vi "test_DiscoveryServiceNotRunning_LaunchDiscoveryService_DiscoveryServiceStarted.vi"(8 "error in":errorcluster) -> (0 "error out":errorcluster, 2 "result":string, 3 "pass":bool)   [LabVIEW 2020, in "MeasurementServerTests.lvlib" / "Discovery Tests.lvlib"]
uses:
  Discovery Tests.lvlib
  Runtime/MeasurementLink Discovery V1/MeasurementLink Discovery V1.lvlib
  MeasurementServerTests.lvlib
  Runtime/MeasurementLink Discovery V1/TypeDefs/gRPC Client Cache FGV Action.ctl
  Runtime/MeasurementLink Discovery Client/MeasurementLink Discovery Client.lvlib
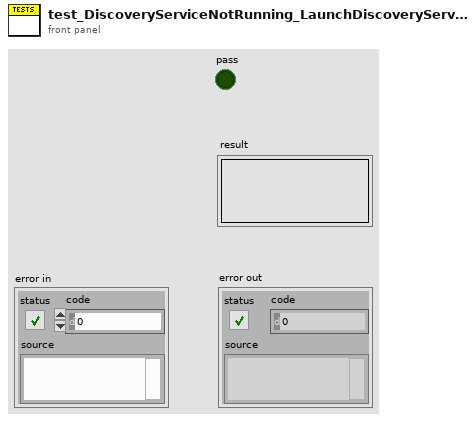
[diagram p1: front panel]
types:
  T1 = typedef "MeasurementLink Discovery V1.lvlib/gRPC Client Cache FGV Action.ctl" = enum16{"Get Client", "Recreate Client"}
  T2 = typedef "grpc-lvsupport-release.lvlib/grpcId.ctl" = u64
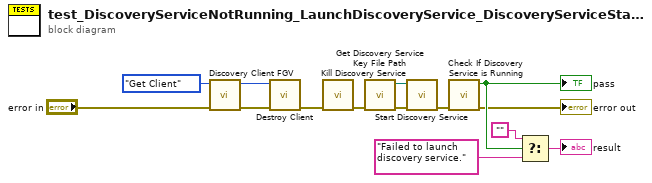
[diagram p0: block diagram]
diagram:
  n1 = call "Discovery Client FGV.vi"("error in"="error in", "action"=gRPC_Client_Cache_FGV_Action."Get Client") -> ("error out"=w4:errorcluster, "grpc client id"=w3:T2)  [unwired: 7 in, 1 out]
  n2 = call "Destroy Client.vi"("error in"=w4, "gRPC ID"=w3) -> ("error out"=w1:errorcluster)  [unwired: 9 in]
  n3 = call "Kill Discovery Service.vi"("error in"=w1) -> ("error out"=w13:errorcluster)  [unwired: 10 in]
  n4 = call "Get Discovery Service Key File Path.vi"("error in"=w13) -> ("error out"=w14:errorcluster, "key file path"=w9:path)  [unwired: 9 in]
  n5 = call "Start Discovery Service.vi"("error in"=w14, "key file path"=w9) -> ("error out"=w8:errorcluster)  [unwired: 9 in]
  n6 = call "Check If Discovery Service is Running.vi"("error in"=w8) -> ("error out"=→"error out":errorcluster, "discovery service running?"=w7:bool)  [unwired: 9 in]
  "pass" <- w7
  n7 = Select(t="", s=w7, f="Failed to launch discovery service.") -> (s? t:f=→"result":string)
